vi "External Transition.vi"(8 "error in (no error)":errorcluster, 9 "Timeout Period in ms (-1, never)":i32=-1, 10 "Target State":refnum<class "_State Machine Actor.lvclass">, 11 "_State Machine Actor in":refnum<class "_State Machine Actor.lvclass">) -> (0 "error out":errorcluster, 3 "_State Machine Actor out":refnum<class "_State Machine Actor.lvclass">)   [LabVIEW 2024]
uses:
  _State Machine Actor.lvclass
  _State Machine Actor.lvclass/_State Machine Actor.ctl
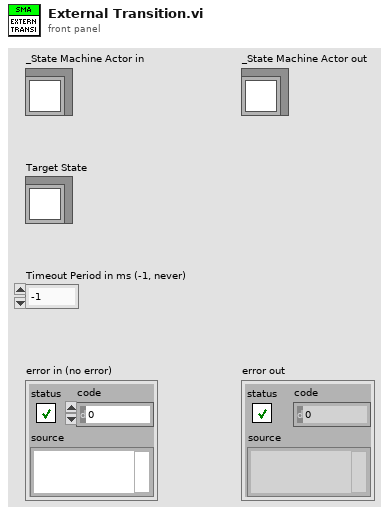
[diagram p1: front panel]
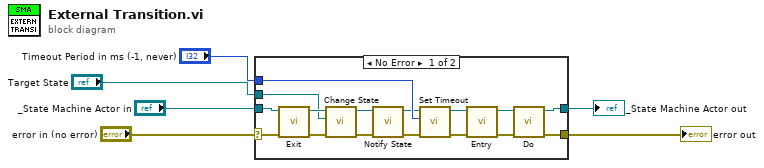
[diagram p0: block diagram]
diagram:
  n1 = case shown="No Error" "error in (no error)" {
    selector: "error in (no error)" -> [w18 w24]
    tunnel: [w16 w24] -> w5
    tunnel: [w20 w23] -> w3
    tunnel: "_State Machine Actor in" -> [w19 w23]
    tunnel: "Target State" -> [w17 _]
    tunnel: "Timeout Period in ms (-1, never)" -> [w13 _]
    frame No Error {
      n2 = call-dynamic "Exit.vi"("error in (no error)"=w18, "State Machine Actor in"=w19) -> ("error out"=w21:errorcluster, "State Machine Actor out"=w22:refnum<class "_State Machine Actor.lvclass">)  [unwired: 8 in]
      n3 = call-dynamic "Change State.vi"("error in (no error)"=w21, "Target State"=w17, "_State Machine Actor in"=w22) -> ("error out"=w11:errorcluster, "_State Machine Actor out"=w12:refnum<class "_State Machine Actor.lvclass">)  [unwired: 7 in]
      n4 = call "Notify State.vi"("error in (no error)"=w11, "_State Machine Actor in"=w12) -> ("error out"=w8:errorcluster, "_State Machine Actor out"=w10:refnum<class "_State Machine Actor.lvclass">)  [unwired: 8 in]
      n5 = call "Set Timeout.vi"("error in (no error)"=w8, "Timeout Period in ms (-1, never)"=w13, "_State Machine Actor in"=w10) -> ("error out"=w14:errorcluster, "_State Machine Actor out"=w15:refnum<class "_State Machine Actor.lvclass">)  [unwired: 7 in]
      n6 = call-dynamic "Entry.vi"("error in (no error)"=w14, "State Machine Actor in"=w15) -> ("error out"=w7:errorcluster, "State Machine Actor out"=w9:refnum<class "_State Machine Actor.lvclass">)  [unwired: 8 in]
      n7 = call-dynamic "Do.vi"("error in (no error)"=w7, "_State Machine Actor in"=w9) -> ("error out"=w16:errorcluster, "_State Machine Actor out"=w20:refnum<class "_State Machine Actor.lvclass">)  [unwired: 8 in]
    }
    frame Error {
    }
  }
  "error out" <- w5
  "_State Machine Actor out" <- w3
